vi "SSL Detection Frame Balls Estimator.vi"(5 "Time Stamp":timestamp, 7 "Life Time":dbl=1.0, 11 "Balls":T1[](array[typedef])) -> (3 "Est balls":T1[](array[typedef]))   [LabVIEW 2018]
uses:
  Controls/SSL Detection Ball.ctl
  <vilib>/Analysis/Matrix/Datatypes/RealMatrix.ctl
  <vilib>/Analysis/Matrix/NI_Matrix.lvlib
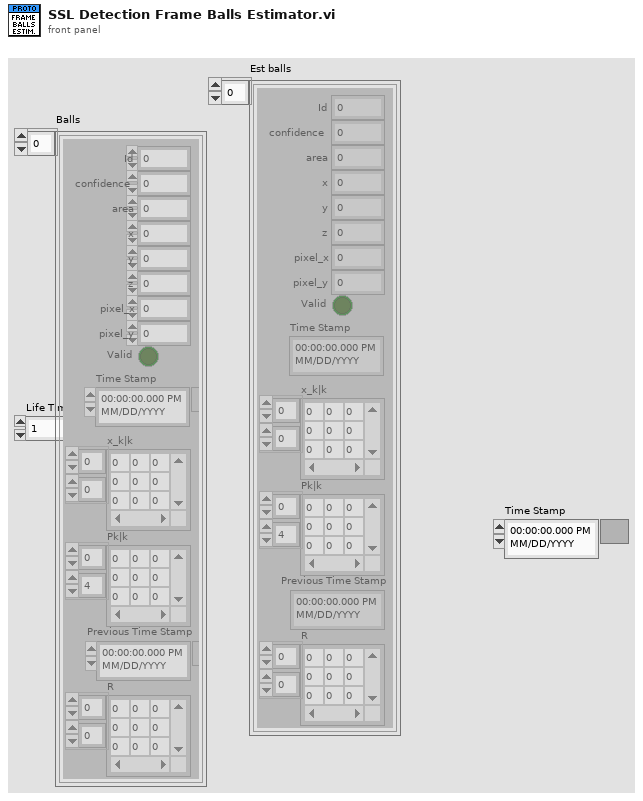
[diagram p1: front panel]
types:
  T1 = typedef "SSL Detection Ball.ctl" = cluster{"x":sgl, "area":u32, "confidence":sgl, "y":sgl, "z":sgl, "pixel_x":sgl, "pixel_y":sgl, "Valid":bool, "Time Stamp":timestamp, "x_k|k":T2, "Pk|k":T2, "Id":u32, "Previous Time Stamp":timestamp, "R":T2}
  T2 = typedef "NI_Matrix.lvlib/RealMatrix.ctl" = dbl[][]
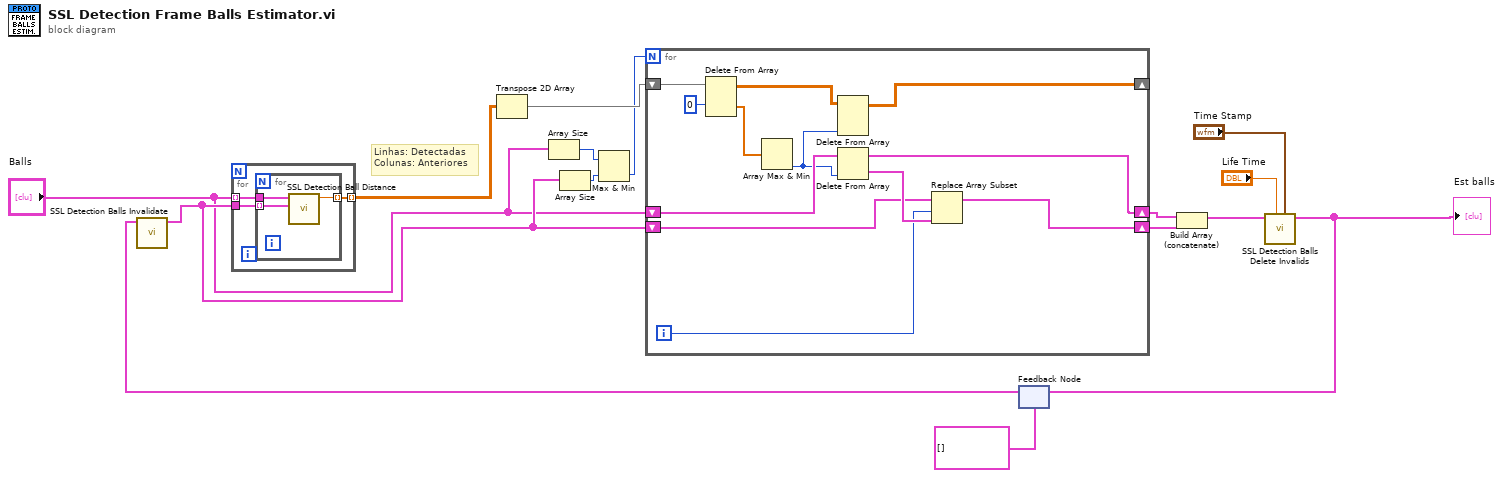
[diagram p0: block diagram]
diagram:
  # "Linhas: Detectadas\nColunas: Anteriores"
  n1 = Array Size(array="Balls") -> (size(s)=w9:i32)
  n2 = feedback #1(T1[] [] ("Balls Out")) -> (w5:T1[])
  n3 = call "SSL Detection Balls Invalidate.vi"("Value"=w5) -> ("Array"=w13:T1[])  [unwired: 10 in]
  n4 = for {
    tunnel: "Balls" -> [w18] mode=indexing
    tunnel: w13 -> [w17]
    tunnel: [w16] -> w15 mode=indexing
    n5 = for {
      tunnel: w18 -> [w21]
      tunnel: w17 -> [w20] mode=indexing
      tunnel: [w19] -> w16 mode=indexing
      n6 = call "SSL Detection Ball Distance.vi"("Detection Ball"=w20, "Detection Ball 2"=w21) -> ("norm"=w19:dbl)  [unwired: 9 in]
    }
  }
  n7 = Transpose 2D Array(2D array=w15) -> (transposed array=w14:dbl[][])
  n8 = Array Size(array=w13) -> (size(s)=w8:i32)
  n9 = Max & Min(x=w9, y=w8) -> (min(x,y)=w7:i32)  [unwired: 1 out]
  n10 = for {
    N: w7 -> [_]
    shift-right: [w27] -> w11
    shift-left: w13 -> [w28]
    shift-right: [w24] -> _
    shift-left: w14 -> [w33]
    shift-right: [w22] -> w12
    shift-left: "Balls" -> [w30]
    i -> [w26]
    n11 = Delete From Array(array=w33, index (row)=0) -> (deleted portion=w31:dbl[], array with subset deleted=w25:dbl[][])  [unwired: 2 in]
    n12 = Array Max & Min(array=w31) -> (min index (indices)=w23:i32)  [unwired: 3 out]
    n13 = Delete From Array(array=w25, index (col)=w23) -> (array with subset deleted=w24:dbl[][])  [unwired: 2 in, 1 out]
    n14 = Delete From Array(array=w30, index=w23) -> (deleted portion=w29:T1, array with subset deleted=w22:T1[])  [unwired: 1 in]
    n15 = Replace Array Subset(array=w28, new element=w29, index=w26) -> (w27:T1[])
  }
  n16 = Build Array (concatenate)(w12, w11) -> (w10:T1[])
  n17 = call "SSL Detection Balls Delete Invalids.vi"("Now"="Time Stamp", "Life Time"="Life Time", "Balls In"=w10) -> ("Balls Out"=w1:T1[])  [unwired: 8 in]
  "Est balls" <- w1
  n18 = feedback-in #1(w1) -> ()
